vi "Fetch Waveform Core.vi"(0 "CS++Scope":refnum<class "CS++Scope.lvclass">, 1 "channel name (\"CHANNEL1\")":string="CHANNEL1", 2 "waveform size (0)":i32=1000, 5 "error in (no error)":errorcluster) -> (14 "CS++Scope out":refnum<class "CS++Scope.lvclass">, 15 "actual points":i32, 16 "initial x":dbl[unit] format="%^.2e", 17 "x increment":dbl[unit] format="%^.2e", 18 "waveform array":dbl[unit][](array[numeric]) format="%.3f", 19 "error out":errorcluster)   [LabVIEW 2015, in "CS++Scope.lvlib" / "CS++Scope.lvclass"]
doc: "This VI returns the waveform the oscilloscope acquires for the channel you specify. The waveform is from an acquisition that you initiate prior to calling this VI.\n\nYou use the IviScope Initiate Acquisition VI to start an acquisition on the channels that you enable with the IviScope Configure Channel VI. The oscilloscope acquires waveforms for the enabled channels concurrently. You use the IviScope Acquisition Status VI to determine when the acquisition is complete. You must call this VI separately for each enabled channel to obtain the waveforms.\n\nYou can call the IviScope Read Waveform VI instead of the IviScope Initiate Acquisition VI. The IviScope Read Waveform VI starts an acquisition on all enabled channels, waits for the acquisition to complete, and returns the waveform for the channel you specify. You call this VI to obtain the waveforms for each of the remaining channels.\n\nNotes:\n\n(1) After this VI executes, each element in the Waveform Array parameter is either a voltage or a value indicating that the oscilloscope could not sample a voltage.\n\n(2) You configure the interpolation method the oscilloscope uses with the IviScope Configure Interpolation [I] VI. If you disable interpolation, the oscilloscope does not interpolate points in the waveform. If the oscilloscope cannot sample a value for a point in the waveform, the driver sets the corresponding element in the Waveform Array to an IEEE defined NaN (Not a Number) value and the VI returns IVISCOPE_WARN_INVALID_WFM_ELEMENT (0x3FFA2001). \n\n(3) You can test a waveform value for an invalid value condition by calling the IviScope Is Invalid Waveform Element VI.\n\n(4) This VI does not check the instrument status. Typically, you call this VI only in a sequence of calls to other low-level driver VIs. The sequence performs one operation. You use the low-level VIs to optimize one or more aspects of interaction with the instrument. If you want to check the instrument status, call the IviScope Error-Query VI at the conclusion of the sequence.\n\n(5) The class driver returns a simulated waveform when this\nVI is called and the IviScope>>Inherent IVI Settings>>User Options>>Simulate property is set to TRUE and the IviScope>>Inherent IVI Settings>>User Options>>Use Specific Simulation property is set to FALSE. For information on how to configure a simulated waveform, refer to the online help manual."
uses:
  CS++Scope.lvclass
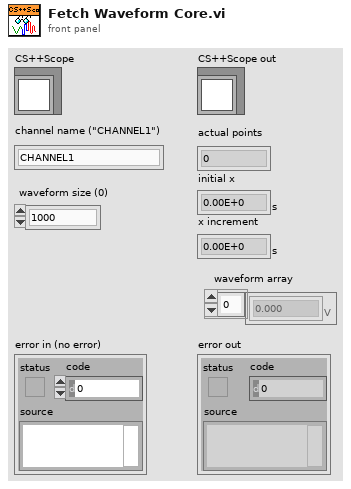
[diagram p1: front panel]
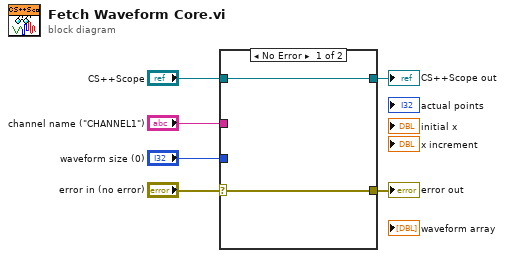
[diagram p0: block diagram]
diagram:
  n1 = case shown="No Error" "error in (no error)" {
    selector: "error in (no error)" -> [w7 w10]
    tunnel: [w7 w10] -> w5
    tunnel: [w8 w9] -> w2
    tunnel: "CS++Scope" -> [w8 w9]
    tunnel: "channel name (\"CHANNEL1\")" -> [_ _]
    tunnel: "waveform size (0)" -> [_ _]
    frame No Error {
    }
    frame Error {
    }
  }
  "error out" <- w5
  "CS++Scope out" <- w2
